vi "MGI Scan From String (CSG).vi"(7 "format string":string="%g", 8 "Default CSG[]":csg, 9 "error in (no error)":errorcluster, 10 "initial scan location":u32, 11 "String In":string) -> (0 "CSG[] Out":csg, 1 "error out":errorcluster, 2 "offset past scan":i32, 3 "Remaining String":string)   [LabVIEW 2016]
doc: "This PolyVI handles scan from string for special datatypes.\n\nAuthored by Shawn Walpole\nsupport@mooregoodideas.com\nwww.mooregoodideas.com\n\nCopyright (c) 2010, Moore Good Ideas, Inc.\n\nAll rights reserved.\n\nRedistribution and use in source and binary forms, with or without modification, are permitted provided that the following conditions are met:\n\n * Redistributions of source code must retain the above copyright notice, this list of conditions and the following disclaimer.\n * Redistributions in binary form must reproduce the above copyright notice, this list of conditions and the following disclaimer in the documentation and/or other materials provided with the distribution.\n * Neither the name of Moore Good Ideas, Inc. nor the names of its contributors may be used to endorse or promote products derived from this software without specific prior written permission.\n\nTHIS SOFTWARE IS PROVIDED BY THE COPYRIGHT HOLDERS AND CONTRIBUTORS \"AS IS\" AND ANY EXPRESS OR IMPLIED WARRANTIES, INCLUDING, BUT NOT LIMITED TO, THE IMPLIED WARRANTIES OF MERCHANTABILITY AND FITNESS FOR A PARTICULAR PURPOSE ARE DISCLAIMED. IN NO EVENT SHALL THE COPYRIGHT OWNER OR CONTRIBUTORS BE LIABLE FOR ANY DIRECT, INDIRECT, INCIDENTAL, SPECIAL, EXEMPLARY, OR CONSEQUENTIAL DAMAGES (INCLUDING, BUT NOT LIMITED TO, PROCUREMENT OF SUBSTITUTE GOODS OR SERVICES; LOSS OF USE, DATA, OR PROFITS; OR BUSINESS INTERRUPTION) HOWEVER CAUSED AND ON ANY THEORY OF LIABILITY, WHETHER IN CONTRACT, STRICT LIABILITY, OR TORT (INCLUDING NEGLIGENCE OR OTHERWISE) ARISING IN ANY WAY OUT OF THE USE OF THIS SOFTWARE, EVEN IF ADVISED OF THE POSSIBILITY OF SUCH DAMAGE."
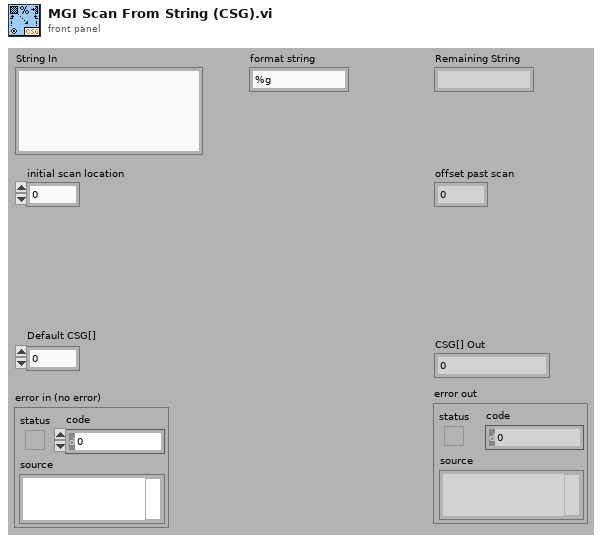
[diagram p1: front panel]
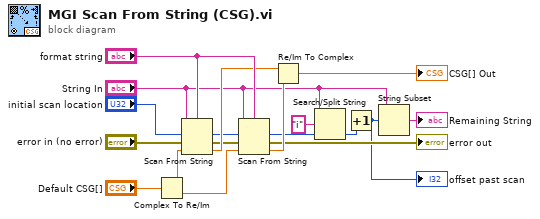
[diagram p0: block diagram]
diagram:
  n1 = Complex To Re/Im(x + iy="Default CSG[]") -> (x=w16:sgl, y=w15:sgl)
  n2 = Scan From String(format string="format string", input string="String In", initial scan location="initial scan location", error in="error in (no error)", default 1=w16) -> (offset past scan=w7:u32, error out=w12:errorcluster, output 1=w14:sgl)  [unwired: 1 out]
  n3 = Scan From String(format string="format string", input string="String In", initial scan location=w7, error in=w12, default 1=w15) -> (offset past scan=w4:u32, error out=→"error out":errorcluster, output 1=w13:sgl)  [unwired: 1 out]
  n4 = Re/Im To Complex(1:w13, 2:w14) -> (0:→"CSG[] Out":csg)
  n5 = Search/Split String(string="String In", search string/char (-)="i", offset (0)=w4) -> (offset of match=w2:i32)  [unwired: 2 out]
  n6 = Increment(x=w2) -> (x+1=w1:i32)
  "offset past scan" <- w1
  n7 = String Subset(string="String In", offset (0)=w1) -> (substring=→"Remaining String":string)  [unwired: 1 in]
